vi "SetMotorWithPID.vi"(5 "DisablePID":bool, 6 "DeadBand":dbl=0.3, 7 "MaxSpeed":dbl=5000.0, 8 "PID gains":T2={"proportional gain (Kc)"=1e-05, "integral time (Ti, min)"=0.0, "derivative time (Td, min)"=0.0} {"proportional gain (Kc)" format="%#_6e"; "integral time (Ti, min)" format="%#_6e"; "derivative time (Td, min)" format="%#_6e"}, 9 "EncoderDevRef":T3={"DevStatus"={"status"=FALSE, "code"=0, "source"=""}, "EncoderIndex"=enum."Invalid", "CounterIndex"=enum."Invalid", "DistancePerCount"=1.0, "Decoding Type"=enum."4x"}, 10 "MotorControlDeviceRef":T7={"DeviceStatus"={"status"=FALSE, "code"=0, "source"=""}, "Type"=enum."PWM", "PWM"={"Digital Module"=enum."Digital Module 1", "PWM Channel"=enum."Invalid", "DeadBand"={"Name"="", "maxPositivePwm"=0, "minPositivePwm"=0, "centerPwm"=0, "maxNegativePwm"=0, "minNegativePwm"=0, "angularRange"=0}}, "CAN"={"Device Number"=0, "Control Mode"=enum."Percent VBus", "Semaphore"=refnum, "Max Vout"=12.0}, "Invert"=FALSE, "TransformRef"=refnum, "InvTransformRef"=refnum}, 11 "Speed":dbl) -> (2 "Debug":T1)   [LabVIEW 2012]
uses:
  <vilib>/Rock Robotics/WPI/MotorControl/WPI_MotorControlDeviceRef.ctl
  <vilib>/Rock Robotics/SystemInterfaces/Typedef/FPGA_TypedefDigitalModule.ctl
  <vilib>/Rock Robotics/SystemInterfaces/DIO/FPGA_DIOPWMChannel.ctl
  <vilib>/Rock Robotics/WPI/PWM/WPI_PWMDeadband.ctl
  <vilib>/Rock Robotics/WPI/CAN/Jaguar/SubVIs/WPI_CANJaguar_ControlMode.ctl
  <vilib>/Rock Robotics/WPI/PWM/WPI_PWMTransform_ConPane.ctl
  <vilib>/Rock Robotics/WPI/Encoder/WPI_EncoderDevRef.ctl
  <vilib>/Rock Robotics/SystemInterfaces/Encoder/FPGA_EncoderIdx.ctl
  <vilib>/Rock Robotics/SystemInterfaces/Counter/FPGA_CounterCtrSystemIndex.ctl
  <vilib>/Rock Robotics/WPI/Encoder/WPI_EncoderType.ctl
  <vilib>/addons/control/pid/pid.llb/PID (DBL).vi
  <vilib>/addons/control/pid/NI_PID_pid.lvlib
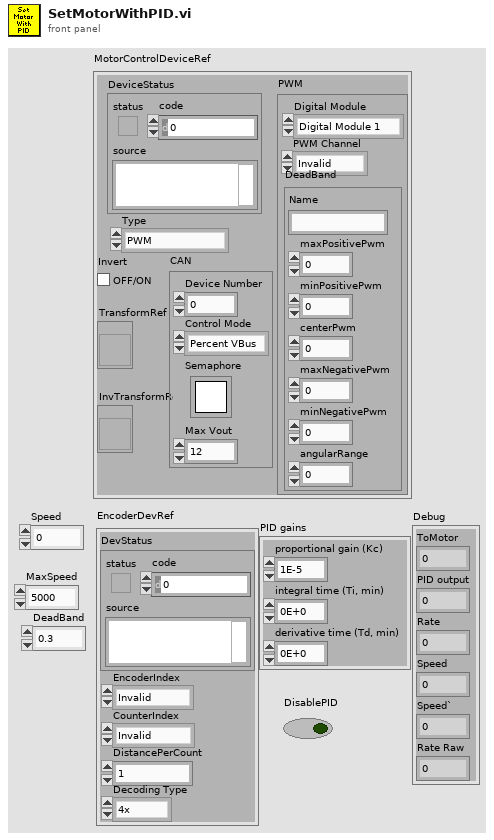
[diagram p1: front panel]
types:
  T1 = cluster{"ToMotor":dbl, "PID output":dbl, "Rate":dbl, "Speed":dbl, "Speed`":dbl, "Rate Raw":dbl}
  T2 = cluster{"proportional gain (Kc)":dbl, "integral time (Ti, min)":dbl, "derivative time (Td, min)":dbl}
  T3 = typedef "WPI_EncoderDevRef.ctl" = cluster{"DevStatus":errorcluster, "EncoderIndex":T4, "CounterIndex":T5, "DistancePerCount":dbl, "Decoding Type":T6}
  T4 = typedef "FPGA_EncoderIdx.ctl" = enum8{"Enc 0", "Enc 1", "Enc 2", "Enc 3", "Invalid"}
  T5 = typedef "FPGA_CounterCtrSystemIndex.ctl" = enum8{"Ctr 0", "Ctr 1", "Ctr 2", "Ctr 3", "Ctr 4", "Ctr 5", "Ctr 6", "Ctr 7", "Invalid"}
  T6 = typedef "WPI_EncoderType.ctl" = enum16{"1x", "2x", "4x"}
  T7 = typedef "WPI_MotorControlDeviceRef.ctl" = cluster{"DeviceStatus":errorcluster, "Type":enum16{"PWM", "CAN"}, "PWM":cluster{"Digital Module":T8, "PWM Channel":T9, "DeadBand":T10}, "CAN":cluster{"Device Number":u8, "Control Mode":T11, "Semaphore":T12, "Max Vout":dbl}, "Invert":bool, "TransformRef":T13, "InvTransformRef":T13}
  T8 = typedef "FPGA_TypedefDigitalModule.ctl" = enum16{"Digital Module 1", "Digital Module 2"}
  T9 = typedef "FPGA_DIOPWMChannel.ctl" = enum8{"PWM 1", "PWM 2", "PWM 3", "PWM 4", "PWM 5", "PWM 6", "PWM 7", "PWM 8", "PWM 9", "PWM 10", "Invalid"}
  T10 = typedef "WPI_PWMDeadband.ctl" = cluster{"Name":string, "maxPositivePwm":i32, "minPositivePwm":i32, "centerPwm":i32, "maxNegativePwm":i32, "minNegativePwm":i32, "angularRange":u16}
  T11 = typedef "WPI_CANJaguar_ControlMode.ctl" = enum8{"Percent VBus", "Current", "Speed", "Position", "Voltage"}
  T12 = typedef "Semaphore RefNum" = refnum<k1>
  T13 = typedef "WPI_PWMTransform_ConPane.ctl" = refnum<vi>
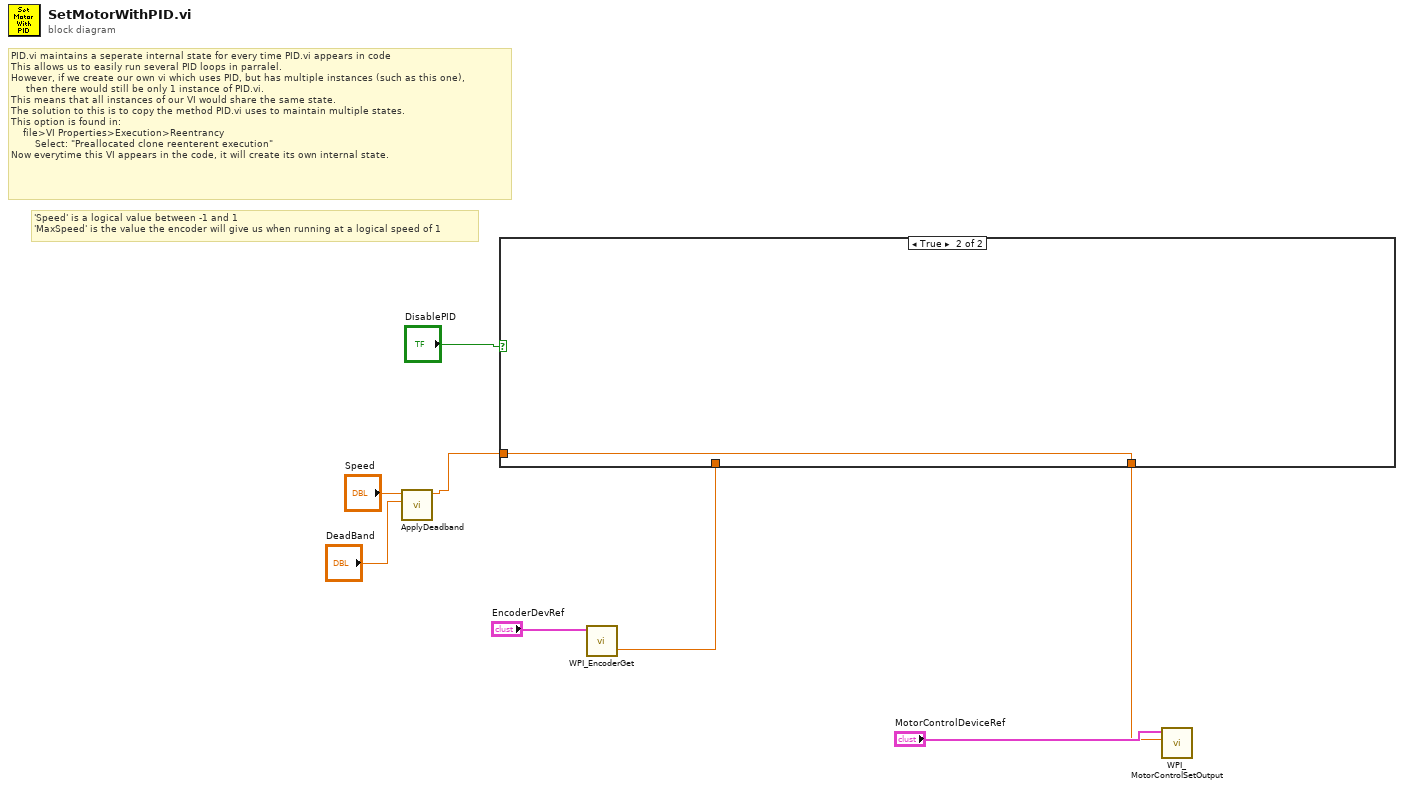
[diagram p0: block diagram]
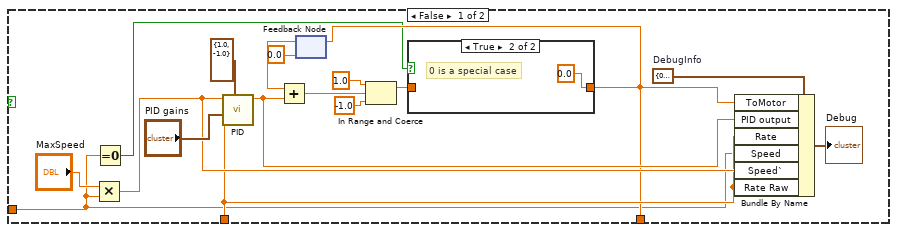
[diagram p2: hidden frame]
diagram:
  # "PID.vi maintains a seperate internal state for every time PID.vi appears in code\nThis allows us to easily run several PID loops in parralel.\nHowever, if we create our own vi which uses PID, but has multiple instances (such as this one), \n     then there would still be only 1 instance of PID.vi.\nThis means that all instances of our VI would share the same state.\nThe solution to this is to copy the method PID.vi uses to maintain multiple states.\nThis option is found in:\n    file>VI Properties>Execution>Reentrancy \n        Select: \"Preallocated clone reenterent execution\"\nNow everytime this VI appears in the code, it will create its own internal state."
  # "'Speed' is a logical value between -1 and 1\n'MaxSpeed' is the value the encoder will give us when running at a logical speed of 1"
  n1 = call "ApplyDeadband.vi"("Deadband"="DeadBand", "Value"="Speed") -> ("Value`"=w2:dbl)  [unwired: 9 in]
  n2 = call <vilib>:"WPI_EncoderGet.vi"("EncoderDevRef"="EncoderDevRef") -> ("Rate"=w6:dbl)  [unwired: 5 in, 5 out]
  n3 = case shown="True" "DisablePID" {
    tunnel: w6 -> [w13 _]
    tunnel: [w11 w28] -> w3
    tunnel: w2 -> [w9 w28]
    frame False {
      w17 = T1 {"ToMotor"=0.0, "PID output"=0.0, "Rate"=0.0, "Speed"=0.0, "Speed`"=0.0, "Rate Raw"=0.0}  # DebugInfo
      n4 = Multiply(x="MaxSpeed", y=w9) -> (x*y=w15:dbl)
      n5 = Equal To 0?(x=w9) -> (x = 0?=w10:bool)
      n6 = call-poly <vilib>:"PID.vi"("output range"=cluster{"output high":dbl, "output low":dbl} {"output high"=1.0, "output low"=-1.0}, "PID gains"="PID gains", "process variable"=w13, "setpoint"=w15) -> ("output"=w16:dbl)  [unwired: 6 in, 1 out]
      n7 = feedback #1(0.0) -> (w24:dbl)
      n8 = Add(x=w24, y=w16) -> (x+y=w23:dbl)
      n9 = In Range and Coerce(upper limit=1.0, x=w23, lower limit=-1.0) -> (coerced(x)=w12:dbl)  [unwired: 1 out]
      n10 = case shown="True" w10 {
        tunnel: w12 -> [w26 _]
        tunnel: [w26 0.0 ("upper limit")] -> w11
        frame False {
        }
        frame True {
          # "0 is a special case"
        }
      }
      n11 = feedback-in #1(w11) -> ()
      n12 = Bundle By Name(cluster=w17, "ToMotor"=w11, "PID output"=w16, "Rate"=w13, "Speed"=w9, "Speed`"=w15, "Rate Raw"=w13) -> (→"Debug":T1)
    }
    frame True {
    }
  }
  n13 = call <vilib>:"WPI_MotorControlSetOutput.vi"("Output"=w3, "MotorControlDevRef"="MotorControlDeviceRef") -> ()  [unwired: 7 in, 3 out]
